vi "String to character Array.vi"(11 "String":string) -> (3 "Array":string[](array[string]))   [LabVIEW 2016, in "Printing.lvlib"]
uses:
  Printing/Printing.lvlib
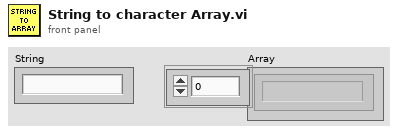
[diagram p1: front panel]
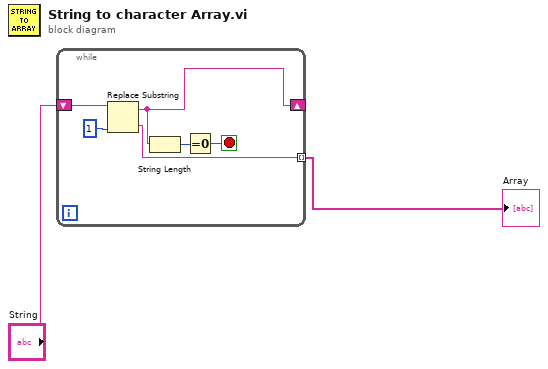
[diagram p0: block diagram]
diagram:
  n1 = while {
    shift-right: [w6] -> _
    shift-left: "String" -> [w7]
    tunnel: [w3] -> w2 mode=indexing
    stop <- w4 stop-if-true
    n2 = Replace Substring(2:1 ("length (len. of substring)"), 5:w7) -> (0:w3:string, 1:w6:string)  [unwired: 2 in]
    n3 = String Length(string=w6) -> (length=w5:i32)
    n4 = Equal To 0?(x=w5) -> (x = 0?=w4:bool)
  }
  "Array" <- w2
